vi "FindTableChangeBlock.vi"(9 "Mode Index":i32=2, 10 "New Array":string[][](array[string])=[["", "", "", "", "", ""], ["", "", "", "", "", ""], ["", "", "", "", "", ""], ["", "", "", "", "", ""], ["", "", "", "", "", ""], ["", "", "", "", "", ""], ["", "", "", "", "", ""]], 11 "Old Array":string[][](array[string])=[["", "", "", "", "", ""], ["", "", "", "", "", ""], ["", "", "", "", "", ""], ["", "", "", "", "", ""], ["", "", "", "", "", ""], ["", "", "", "", "", ""], ["", "", "", "", "", ""]]) -> (0 "Size mismatch?":bool, 1 "Mode change?":bool, 2 "changed? subarray":bool[][](array[boolean]), 3 "Change start":T1)   [LabVIEW 2013]
doc: "Compare Old/New Array and determine block locatation and size of difference, indicating whether that change includes \"Mode Index\" by setting \"Mode change?\" If Old and New Array are not the same size, \"SizeMismatch?\" is set. In this case, the output change block is only for the overlap of Old and New.\n\nIf no change is found, Change start will be (-1,-1) while change size will be (0,0).\n\nWhile nearly all changes to SetList table are block-wise, this function returns a block which encapsulates all (non-contiguous, ragged) changes by a single block."
uses:
  <vilib>/Utility/miscctls.llb/LVRowAndColumnTypeDef.ctl
panel:
  out "runtime (ms)":u32
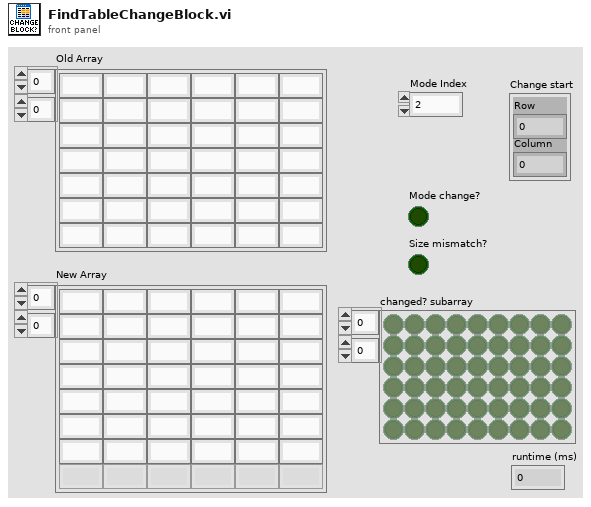
[diagram p1: front panel]
types:
  T1 = typedef "LVRowAndColumnTypeDef.ctl" = cluster{"Row":i32, "Column":i32}
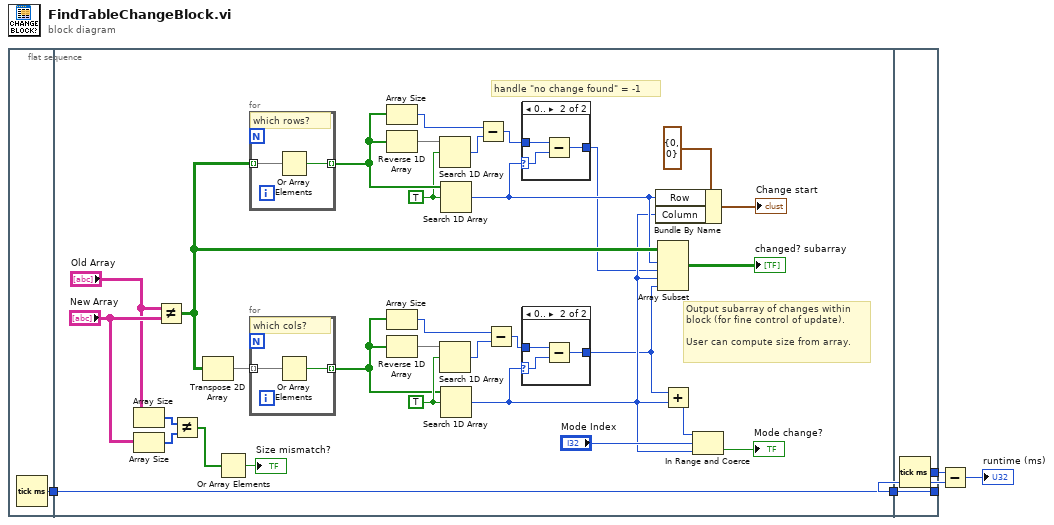
[diagram p0: block diagram]
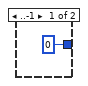
[diagram p2: hidden frame]
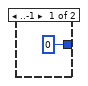
[diagram p3: hidden frame]
diagram:
  n1 = flat-sequence {
    tunnel: [w6] -> w5
    tunnel: w5 -> [w20]
    tunnel: [w20] -> w2
    tunnel: [w51] -> w3
    tunnel: w2 -> [w50]
    tunnel: [w50] -> w1
    frame #0 {
      n2 = Tick Count (ms)() -> (millisecond timer value=w6:u32)
    }
    frame #1 {
      w29 = TRUE ("element")
      w35 = TRUE ("element")
      # "Output subarray of changes within\nblock (for fine control of update).\n\nUser can compute size from array."
      # "handle \"no change found\" = -1"
      n3 = Array Size(array="Old Array") -> (size(s)=w17:i32[])
      n4 = Array Size(array="New Array") -> (size(s)=w16:i32[])
      n5 = Not Equal?(x="Old Array", y="New Array") -> (x != y?=w12:bool[][])
      n6 = Not Equal?(x=w17, y=w16) -> (x != y?=w14:bool[])
      n7 = Transpose 2D Array(2D array=w12) -> (transposed array=w26:bool[][])
      n8 = Or Array Elements(Boolean array=w14) -> (logical OR=→"Size mismatch?":bool)
      n9 = for {
        tunnel: w12 -> [w49] mode=indexing
        tunnel: [w48] -> w36 mode=indexing
        # "which rows?"
        n10 = Or Array Elements(Boolean array=w49) -> (logical OR=w48:bool)
      }
      n11 = for {
        tunnel: w26 -> [w47] mode=indexing
        tunnel: [w46] -> w28 mode=indexing
        # "which cols?"
        n12 = Or Array Elements(Boolean array=w47) -> (logical OR=w46:bool)
      }
      n13 = Array Size(array=w36) -> (size(s)=w33:i32)
      n14 = Reverse 1D Array(array=w36) -> (reversed array=w37:bool[])
      n15 = Array Size(array=w28) -> (size(s)=w31:i32)
      n16 = Reverse 1D Array(array=w28) -> (reversed array=w27:bool[])
      n17 = Search 1D Array(1D array=w37, element=w35) -> (index of element=w34:i32)  [unwired: 1 in]
      n18 = Search 1D Array(1D array=w27, element=w29) -> (index of element=w30:i32)  [unwired: 1 in]
      n19 = Search 1D Array(1D array=w36, element=w35) -> (index of element=w11:i32)  [unwired: 1 in]
      n20 = Search 1D Array(1D array=w28, element=w29) -> (index of element=w10:i32)  [unwired: 1 in]
      n21 = Subtract(x=w33, y=w34) -> (x-y=w32:i32)
      n22 = Subtract(x=w31, y=w30) -> (x-y=w13:i32)
      n23 = case shown="0.." w11 {
        selector: w11 -> [_ w43]
        tunnel: w32 -> [_ w45]
        tunnel: [0 w44] -> w9
        frame ..-1 {
        }
        frame 0.. {
          n24 = Subtract(x=w45, y=w43) -> (x-y=w44:i32)
        }
      }
      n25 = case shown="0.." w10 {
        selector: w10 -> [_ w39]
        tunnel: w13 -> [_ w41]
        tunnel: [0 w40] -> w8
        frame ..-1 {
        }
        frame 0.. {
          n26 = Subtract(x=w41, y=w39) -> (x-y=w40:i32)
        }
      }
      n27 = Bundle By Name(cluster=T1 {"Row"=0, "Column"=0} ("Change size"), "Row"=w11, "Column"=w10) -> (→"Change start":T1)
      n28 = Array Subset(array=w12, index (row)=w11, length (row)=w9, index (col)=w10, length (col)=w8) -> (→"changed? subarray":bool[][])
      n29 = Add(x=w8, y=w10) -> (x+y=w22:i32)
      n30 = In Range and Coerce(upper limit=w22, x="Mode Index", lower limit=w10) -> (In Range?=→"Mode change?":bool)  [unwired: 1 out]
    }
    frame #2 {
      n31 = Tick Count (ms)() -> (millisecond timer value=w51:u32)
    }
  }
  n32 = Subtract(x=w3, y=w1) -> (x-y=→"runtime (ms)":u32)
